vi "setGains.vi"(0 "Interface in":T1, 5 "gains":T2 {"proportional gain" step=0.125}, 11 "error in (no error)":errorcluster) -> (4 "Interface out":T1, 15 "error out":errorcluster)   [LabVIEW 2017, in "BuckBoostInterface.lvlib"]
uses:
  BuckBoostInterface.lvlib
  <vilib>/rvi/Analysis/control/PID/Typedef/niFpgaPID_PIGains.ctl
  Interface.ctl
  <instrlib>/_niInstr/Instruction Framework/v1/Host/Instruction Target/niInstr Instruction Target v1 Host.lvclass
  <instrlib>/_niInstr/Instruction Framework/v1/Host/Instruction Framework Context/niInstr Instruction Framework Context v1 Host.lvclass
  <vilib>/NI/JSON Support for LabVIEW/JSON Data Classes/JSON Object/New JSON Object (Empty).vi
  <vilib>/NI/JSON Support for LabVIEW/JSON Data Classes/JSON Object/Insert Key Value Pair (Single).vi
  <vilib>/NI/JSON Support for LabVIEW/JSON Data Classes/JSON Helper/Parsing/Parse Value.vi
  <vilib>/NI/JSON Support for LabVIEW/JSON Data Classes/JSON Helper/To More Specific Type (Object).vi
  <vilib>/NI/JSON Support for LabVIEW/JSON Data Classes/JSON Datatype/JSON Null.lvclass
  <vilib>/NI/JSON Support for LabVIEW/JSON Data Classes/JSON Object/JSON Object.lvclass
  <vilib>/NI/JSON Support for LabVIEW/JSON Data Classes/JSON Helper/JSON Helper.lvclass
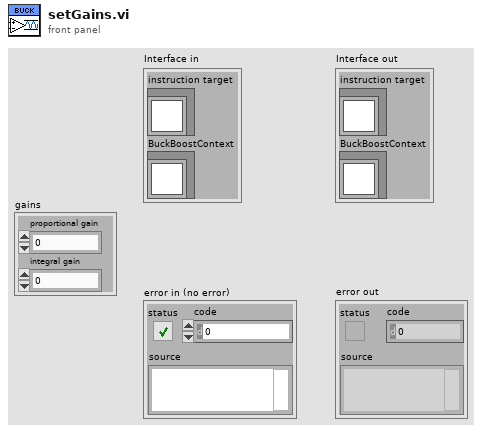
[diagram p1: front panel]
types:
  T1 = typedef "BuckBoostInterface.lvlib/Interface.ctl" = cluster{"instruction target":refnum<class "niInstr Instruction Target v1 Host.lvclass">, "BuckBoostContext":refnum<class "niInstr Instruction Framework Context v1 Host.lvclass">}
  T2 = typedef "niFpgaPID_PIGains.ctl" = cluster{"proportional gain":sgl, "integral gain":sgl}
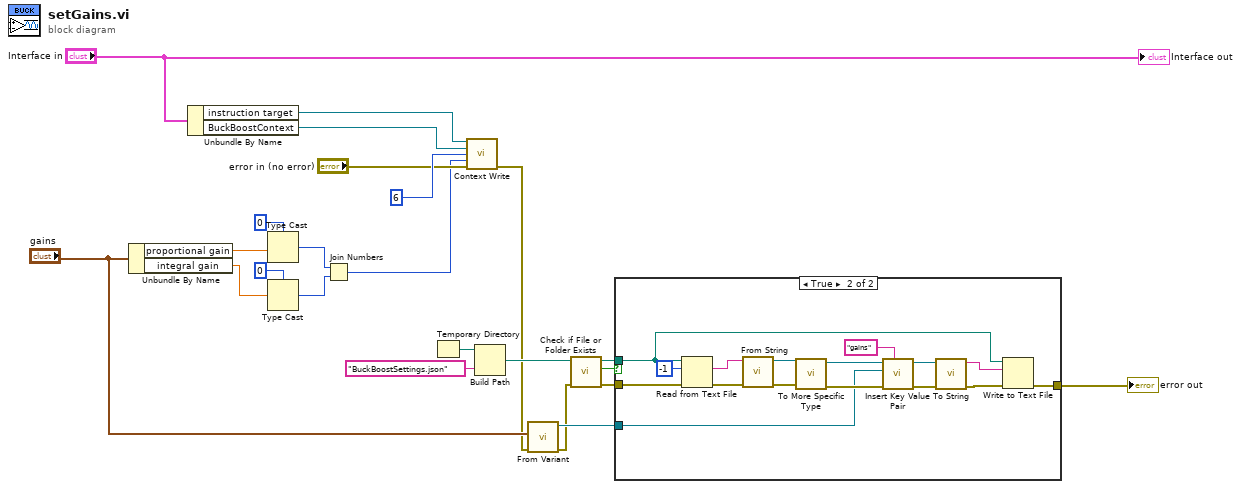
[diagram p0: block diagram]
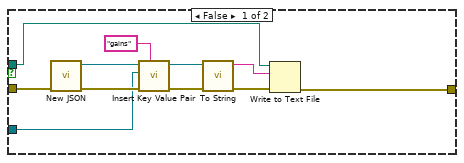
[diagram p2: hidden frame]
diagram:
  n1 = Unbundle By Name("gains") -> ("proportional gain"=w20:sgl, "integral gain"=w23:sgl)
  n2 = Unbundle By Name("Interface in") -> ("instruction target"=w16:refnum<class "niInstr Instruction Target v1 Host.lvclass">, "BuckBoostContext"=w15:refnum<class "niInstr Instruction Framework Context v1 Host.lvclass">)
  n3 = Type Cast(type=u32 0, x=w20) -> (*(type *) &x=w14:u32)
  n4 = Type Cast(type=u32 0, x=w23) -> (*(type *) &x=w13:u32)
  n5 = Join Numbers(hi=w14, lo=w13) -> ((hi.lo)=w12:u64)
  n6 = Temporary Directory() -> (w11:path)
  n7 = call <instrlib>:"Context Write.vi"("instruction target in"=w16, "context in"=w15, "address"=u64 6, "data"=w12, "error in"="error in (no error)") -> ("error out"=w3:errorcluster)  [unwired: 8 in, 2 out]
  n8 = Build Path(base path=w11, name or relative path="BuckBoostSettings.json") -> (appended path=w9:path)
  n9 = call <vilib>:"From Variant.vi"("error in (no error)"=w3, "Variant"="gains") -> ("error out"=w2:errorcluster, "JSON out"=w6:refnum<class "JSON Null.lvclass">)  [unwired: 8 in]
  n10 = call <vilib>:"Check if File or Folder Exists.vi"("error in (no error)"=w2, "path"=w9) -> ("error out"=w4:errorcluster, "file or folder exists?"=w7:bool, "dup path"=w8:path)  [unwired: 7 in]
  n11 = case shown="True" w7 {
    tunnel: w8 -> [w29 w41]
    tunnel: w6 -> [w31 w43]
    tunnel: w4 -> [w34 w42]
    tunnel: [w28 w36] -> w1
    frame False {
      n12 = call-poly <vilib>:"New JSON.vi"("error in (no error)"=w34) -> ("error out"=w32:errorcluster, "JSON Object out"=w33:refnum<class "JSON Object.lvclass">)  [unwired: 9 in]
      n13 = call-poly <vilib>:"Insert Key Value Pair.vi"("key"="gains", "error in (no error)"=w32, "value"=w31, "JSON Object in"=w33) -> ("error out"=w27:errorcluster, "JSON Object out"=w24:refnum<class "JSON Object.lvclass">)  [unwired: 5 in, 1 out]
      n14 = call-dynamic "To String.vi"("error in (no error)"=w27, "JSON Object in"=w24) -> ("error out"=w26:errorcluster, "String"=w25:string)  [unwired: 8 in]
      n15 = Write to Text File(file (use dialog)=w29, text=w25, error in=w26) -> (error out=w28:errorcluster)  [unwired: 1 in, 2 out]
    }
    frame True {
      n16 = Read from Text File(file (use dialog)=w41, count=-1, error in=w42) -> (text=w50:string, error out=w45:errorcluster)  [unwired: 1 in, 2 out]
      n17 = call <vilib>:"From String.vi"("error in (no error)"=w45, "JSON String"=w50) -> ("error out"=w49:errorcluster, "JSON out"=w48:refnum<class "JSON Null.lvclass">)  [unwired: 8 in]
      n18 = call-poly <vilib>:"To More Specific Type.vi"("error in (no error)"=w49, "JSON Datatype in"=w48) -> ("error out"=w46:errorcluster, "JSON Datatype out"=w47:refnum<class "JSON Object.lvclass">)  [unwired: 8 in]
      n19 = call-poly <vilib>:"Insert Key Value Pair.vi"("key"="gains", "error in (no error)"=w46, "value"=w43, "JSON Object in"=w47) -> ("error out"=w38:errorcluster, "JSON Object out"=w40:refnum<class "JSON Object.lvclass">)  [unwired: 5 in, 1 out]
      n20 = call-dynamic "To String.vi"("error in (no error)"=w38, "JSON Object in"=w40) -> ("error out"=w37:errorcluster, "String"=w39:string)  [unwired: 8 in]
      n21 = Write to Text File(file (use dialog)=w41, text=w39, error in=w37) -> (error out=w36:errorcluster)  [unwired: 1 in, 2 out]
    }
  }
  "error out" <- w1
  "Interface out" <- "Interface in"
